vi "Reset Status.vi"(10 "Run Queue":set{string}(c389), 11 "Result Model in":refnum<class "Result Model.lvclass">) -> ()   [LabVIEW 2020, in "Result Model.lvclass"]
uses:
  Result Model.lvclass
  Result Model.lvclass/Result Model.ctl
  Core/Result/Status.ctl
  Core/Result/Result.lvlib
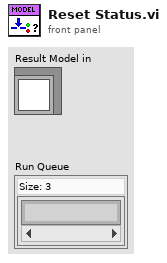
[diagram p1: front panel]
types:
  T1 = typedef "Result.lvlib/Status.ctl" = enum16{"", "Passed", "Failed", "Error", "Skipped", "Setup Error", "Broken", "Teardown Error"}
  T2 = typedef "Result Model.lvclass/Model State.ctl" = cluster{"Run Queue":set{string}, "Test Statuses":map{string, T1}, "Execution Time":map{string, dbl}, "Assertions":map{string, cluster{"Result Type":T3, "Status":T1, "Message":string, "Description":string}[]}}
  T3 = typedef "Result.lvlib/Type.ctl" = enum16{"Method", "Case", "Suite", "Pass", "Fail", "Skip", "Pass if", "Fail if", "Pass if Error", "Fail if Error", "Pass if Equal", "Fail if Equal"}
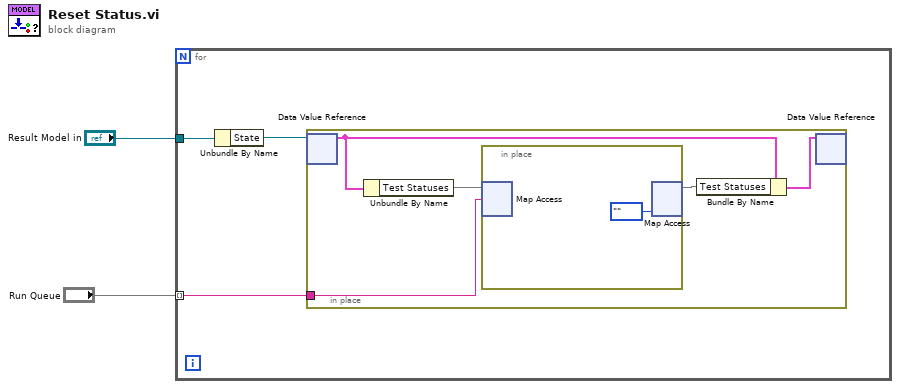
[diagram p0: block diagram]
diagram:
  n1 = for {
    tunnel: "Result Model in" -> [w5]
    tunnel: "Run Queue" -> [w3] mode=indexing
    n2 = Unbundle By Name(w5) -> ("State"=w4:refnum<data-value>)
    n3 = in-place {
      in-place-border: w3 -> [w7]
      n4 = in-place-dvr #1(w4) -> (w9:T2)  [unwired: 1 out]
      n5 = Unbundle By Name(w9) -> ("Test Statuses"=w8:map{string, T1})
      n6 = in-place {
        n7 = in-place-map #2(w8, w7) -> ()  [unwired: 1 in, 2 out]
        n8 = in-place-map #2(Status."" ("value")) -> (w6:map{string, T1})  [unwired: 1 in, 2 out]
      }
      n9 = Bundle By Name(cluster=w9, "Test Statuses"=w6) -> (w10:T2)
      n10 = in-place-dvr #1(w10) -> ()  [unwired: 2 out]
    }
  }
